vi "pre1.vi"() -> ()   [LabVIEW 2020]
panel:
  in  "Select a Channel":dbl
  out "Output Array":dbl[](array[numeric])
  in  "Input Array":dbl[](array[numeric])
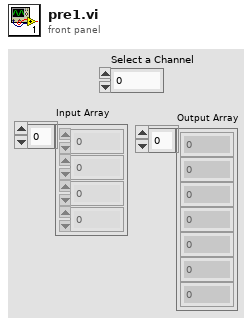
[diagram p1: front panel]
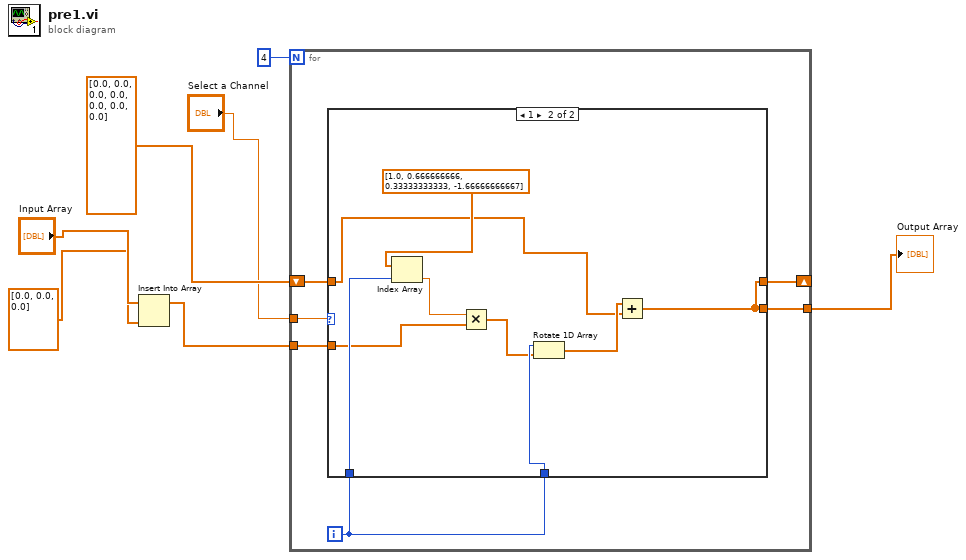
[diagram p0: block diagram]
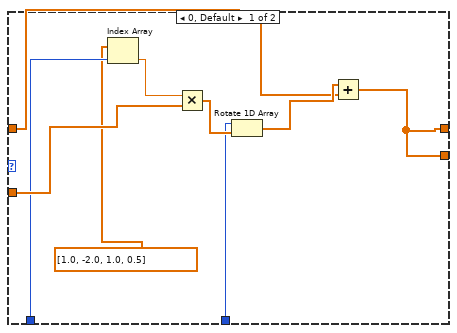
[diagram p2: hidden frame]
diagram:
  n1 = Insert Into Array(array="Input Array", new element=dbl[] [0.0, 0.0, 0.0]) -> (w3:dbl[])  [unwired: 1 in]
  n2 = for {
    N: 4 -> [_]
    tunnel: "Select a Channel" -> [w13]
    shift-right: [w9] -> _
    shift-left: dbl[] [0.0, 0.0, 0.0, 0.0, 0.0, 0.0, 0.0] -> [w12]
    tunnel: [w10] -> w4
    tunnel: w3 -> [w11]
    i -> [w8]
    n3 = case shown="1" w13 {
      tunnel: [w18 w27] -> w10
      tunnel: w8 -> [w20 w31]
      tunnel: w12 -> [w14 w23]
      tunnel: w11 -> [w21 w29]
      tunnel: [w18 w27] -> w9
      tunnel: w8 -> [w16 w26]
      frame 0, Default {
        n4 = Index Array(array=dbl[] [1.0, -2.0, 1.0, 0.5], index=w20) -> (element=w22:dbl)
        n5 = Multiply(x=w22, y=w21) -> (x*y=w17:dbl[])
        n6 = Rotate 1D Array(1:w17, 2:w16) -> (0:w15:dbl[])
        n7 = Add(x=w15, y=w14) -> (x+y=w18:dbl[])
      }
      frame 1 {
        n8 = Index Array(array=dbl[] [1.0, 0.666666666, 0.33333333333, -1.66666666667], index=w31) -> (element=w28:dbl)
        n9 = Multiply(x=w28, y=w29) -> (x*y=w25:dbl[])
        n10 = Rotate 1D Array(1:w25, 2:w26) -> (0:w24:dbl[])
        n11 = Add(x=w24, y=w23) -> (x+y=w27:dbl[])
      }
    }
  }
  "Output Array" <- w4
